vi "Check OS Supports Small Fonts.vi"() -> (3 "os_supports_small_fonts":bool)   [LabVIEW 2021, in "Picture Pixel Fonts.lvlib"]
uses:
  <vilib>/LabVIEW Icon API/Pixel Fonts/Picture Pixel Fonts.lvlib
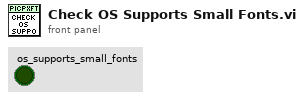
[diagram p1: front panel]
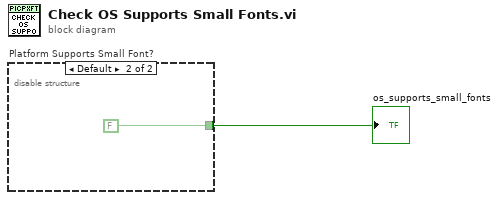
[diagram p0: block diagram]
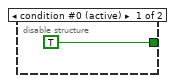
[diagram p2: hidden frame]
diagram:
  n1 = disable-structure "Platform Supports Small Font?" shown="Default" {
    disable-tunnel: [TRUE FALSE] -> w1
    frame condition #0 (active) {
    }
    frame condition #1 {
    }
  }
  "os_supports_small_fonts" <- w1
